vi "ControlFile.vi"(8 "error in (no error)":errorcluster, 10 "Description":string, 11 "Package Builder in":refnum<class "Package Builder.lvclass">) -> (0 "error out":errorcluster, 3 "Package Builder out":refnum<class "Package Builder.lvclass">)   [LabVIEW 2020, in "Package Builder.lvclass"]
uses:
  Package Builder.lvclass
  Package Builder.lvclass/Package Builder.ctl
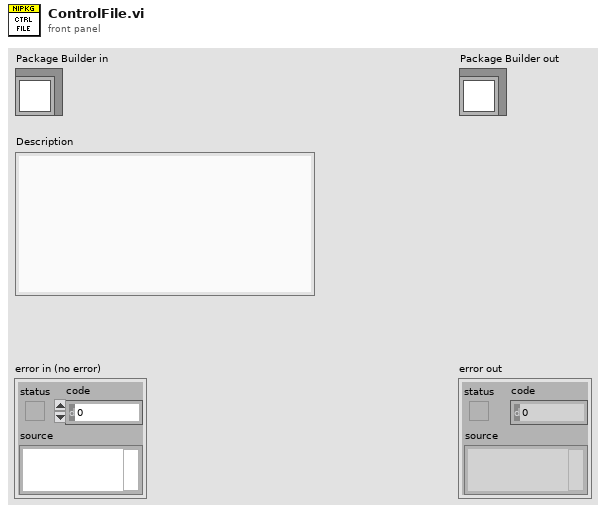
[diagram p1: front panel]
types:
  T1 = enum16{"open", "replace", "create", "open or create", "replace or create", "replace or create with confirmation"}
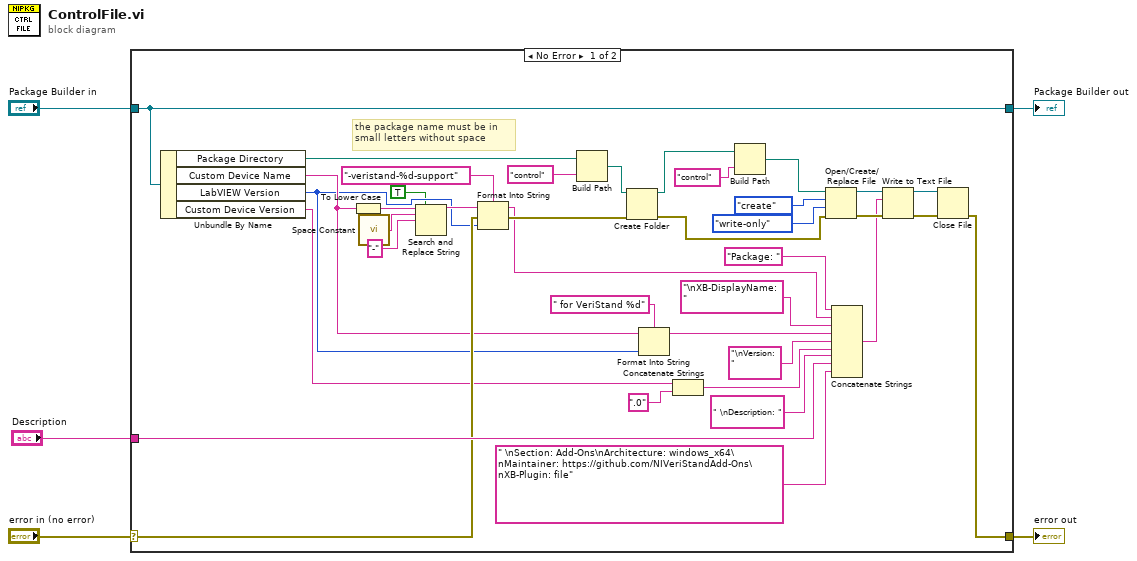
[diagram p0: block diagram]
diagram:
  n1 = case shown="No Error" "error in (no error)" {
    selector: "error in (no error)" -> [w16 w45]
    tunnel: [w25 w45] -> w4
    tunnel: [w27 w44] -> w2
    tunnel: "Package Builder in" -> [w27 w44]
    tunnel: "Description" -> [w24 _]
    frame No Error {
      # "the package name must be in small letters without space"
      n2 = Unbundle By Name(w27) -> ("Package Directory"=w26:path, "Custom Device Name"=w10:string, "LabVIEW Version"=w7:u32, "Custom Device Version"=w14:string)
      n3 = To Lower Case(string=w10) -> (all lower case string=w21:string)
      n4 = call <vilib>:"Space Constant.vi"() -> ("String"=w20:string)
      n5 = Search and Replace String(replace all?=TRUE ("replace all? (F)"), input string=w21, search string=w20, replace string="-" ("replace string (\"\")")) -> (result string=w19:string)  [unwired: 4 in, 3 out]
      n6 = Format Into String(format string="-veristand-%d-support", initial string=w19, error in=w16, w7) -> (resulting string=w12:string, error out=w17:errorcluster)
      n7 = Build Path(base path=w26, name or relative path="control" ("time format string (%c)")) -> (appended path=w43:path)
      n8 = Create Folder(path (use dialog)=w43, error in=w17) -> (created path=w31:path, error out=w29:errorcluster)  [unwired: 1 in, 1 out]
      n9 = Format Into String(format string=" for VeriStand %d", initial string=w10, w7) -> (resulting string=w8:string)  [unwired: 1 in, 1 out]
      n10 = Concatenate Strings(w14, ".0" ("initial string")) -> (w22:string)
      n11 = Build Path(base path=w31, name or relative path="control" ("time format string (%c)")) -> (appended path=w30:path)
      n12 = Open/Create/Replace File(file path (use dialog)=w30, error in=w29, operation (0:open)=T1."create", access (0:read/write)=enum16{"read/write", "read-only", "write-only"}."write-only") -> (refnum out=w36:refnum<file>, error out=w35:errorcluster)  [unwired: 2 in, 1 out]
      n13 = Concatenate Strings("Package: " ("initial string"), w12, "\nXB-DisplayName: " ("initial string"), w8, "\nVersion: " ("initial string"), w22, " \nDescription: " ("initial string"), w24, " \nSection: Add-Ons\nArchitecture: windows_x64\nMaintainer: https://github.com/NIVeriStandAdd-Ons\nXB-Plugin: file" ("initial string")) -> (w28:string)
      n14 = Write to Text File(file (use dialog)=w36, text=w28, error in=w35) -> (refnum out=w37:refnum<file>, error out=w38:errorcluster)  [unwired: 1 in, 1 out]
      n15 = Close File(refnum=w37, error in=w38) -> (error out=w25:errorcluster)  [unwired: 1 out]
    }
    frame Error {
    }
  }
  "error out" <- w4
  "Package Builder out" <- w2
